vi "Performance Vs Average.vi"(10 "Master Calculated Stats":T2(array[cluster]), 11 "Last Week's Calculated Stats":T2(array[cluster])) -> (3 "Last Week's Performance vs Historical Averages":T1(array[cluster]))   [LabVIEW 2020]
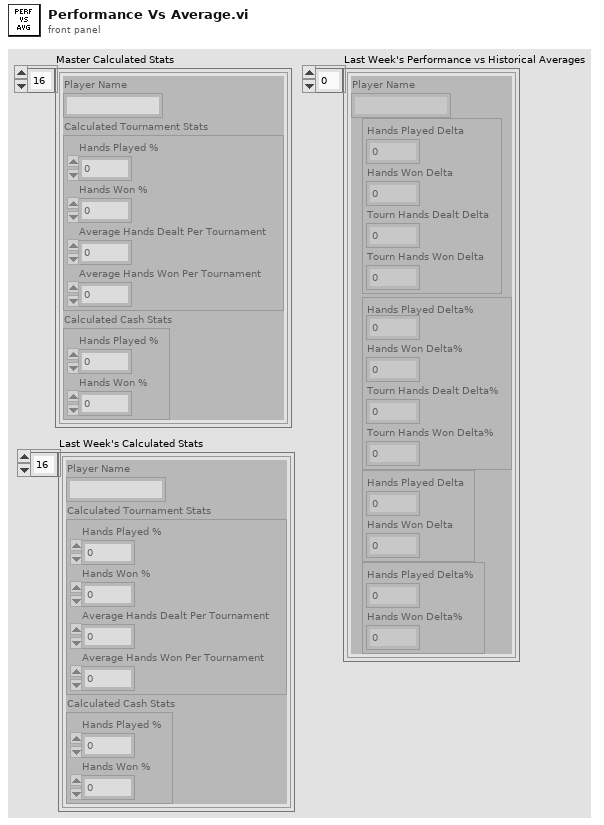
[diagram p1: front panel]
types:
  T1 = cluster{"Player Name":string, cluster{"Hands Played Delta":dbl, "Hands Won Delta":dbl, "Tourn Hands Dealt Delta":dbl, "Tourn Hands Won Delta":dbl}, cluster{"Hands Played Delta%":dbl, "Hands Won Delta%":dbl, "Tourn Hands Dealt Delta%":dbl, "Tourn Hands Won Delta%":dbl}, cluster{"Hands Played Delta":dbl, "Hands Won Delta":dbl}, cluster{"Hands Played Delta%":dbl, "Hands Won Delta%":dbl}}[]
  T2 = cluster{"Player Name":string, "Calculated Tournament Stats":cluster{"Hands Played %":dbl, "Hands Won %":dbl, "Average Hands Dealt Per Tournament":dbl, "Average Hands Won Per Tournament":dbl}, "Calculated Cash Stats":cluster{"Hands Played %":dbl, "Hands Won %":dbl}}[]
  T3 = cluster{"Hands Played %":dbl, "Hands Won %":dbl, "Average Hands Dealt Per Tournament":dbl, "Average Hands Won Per Tournament":dbl}
  T4 = cluster{"[0]":dbl, "[1]":dbl, "[2]":dbl, "[3]":dbl}
  T5 = cluster{"f":string, cluster{"[0]":dbl, "[1]":dbl, "[2]":dbl, "[3]":dbl}, cluster{"[0]":dbl, "[1]":dbl, "[2]":dbl, "[3]":dbl}, cluster{"[0]":dbl, "[1]":dbl}, cluster{"[0]":dbl, "[1]":dbl}}
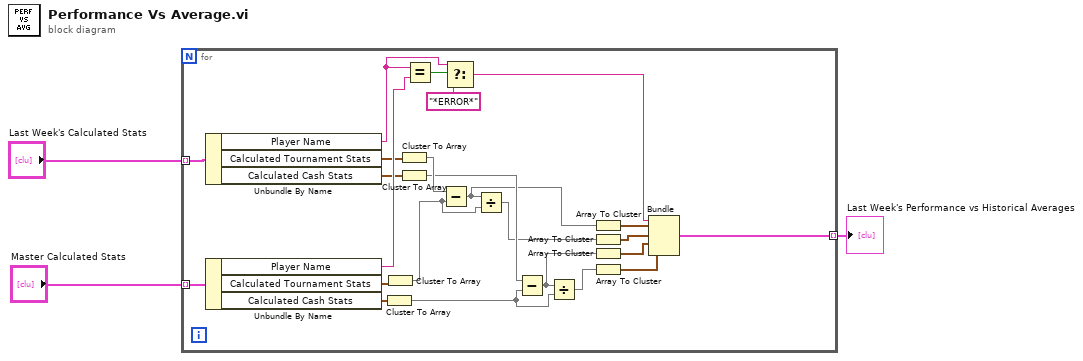
[diagram p0: block diagram]
diagram:
  n1 = for {
    tunnel: "Master Calculated Stats" -> [w26] mode=indexing
    tunnel: "Last Week's Calculated Stats" -> [w27] mode=indexing
    tunnel: [w4] -> w1 mode=indexing
    n2 = Unbundle By Name(w27) -> ("Player Name"=w23:string, "Calculated Tournament Stats"=w19:T3, "Calculated Cash Stats"=w18:cluster{"Hands Played %":dbl, "Hands Won %":dbl})
    n3 = Unbundle By Name(w26) -> ("Player Name"=w25:string, "Calculated Tournament Stats"=w21:T3, "Calculated Cash Stats"=w20:cluster{"Hands Played %":dbl, "Hands Won %":dbl})
    n4 = Cluster To Array(cluster=w20) -> (array=w14:dbl[])
    n5 = Cluster To Array(cluster=w21) -> (array=w15:dbl[])
    n6 = Cluster To Array(cluster=w19) -> (array=w17:dbl[])
    n7 = Cluster To Array(cluster=w18) -> (array=w16:dbl[])
    n8 = Equal?(x=w23, y=w25) -> (x = y?=w24:bool)
    n9 = Subtract(x=w17, y=w15) -> (x-y=w12:dbl[])
    n10 = Select(t=w23, s=w24, f="*ERROR*") -> (s? t:f=w13:string)
    n11 = Divide(x=w12, y=w15) -> (x/y=w10:dbl[])
    n12 = Subtract(x=w16, y=w14) -> (x-y=w8:dbl[])
    n13 = Divide(x=w8, y=w14) -> (x/y=w7:dbl[])
    n14 = Array To Cluster(array=w12) -> (cluster=w11:T4)
    n15 = Array To Cluster(array=w10) -> (cluster=w9:T4)
    n16 = Array To Cluster(array=w8) -> (cluster=w6:cluster{"[0]":dbl, "[1]":dbl})
    n17 = Array To Cluster(array=w7) -> (cluster=w5:cluster{"[0]":dbl, "[1]":dbl})
    n18 = Bundle("f"=w13, w11, w9, w6, w5) -> (w4:T5)  [unwired: 1 in]
  }
  "Last Week's Performance vs Historical Averages" <- w1
